vi "Create Ramp Buffer.vi"(8 "error in (no error)":errorcluster, 10 "initial value":u8, 11 "size":u64=1024) -> (0 "error out":errorcluster, 2 "buffer out":u8[](array[numeric]), 3 "pointer out":refnum<class "Memory.Pointer.Internal.lvclass">)   [LabVIEW 2016, in "Memory Manager Unit Tests.lvclass"]
uses:
  Memory Manager Unit Tests.lvclass
  Library/Classes/Pointer.Internal/Memory.Pointer.Internal.lvclass
  C:/Git/Personal/LabVIEW-Memory-Manager/Source/Library/Classes/Pointer/Memory.Pointer.lvclass
  Library/Classes/Pointer/Memory.Pointer.lvclass/Memory.Pointer.ctl
  Library/Classes/Pointer/Methods/Memory.Pointer.Write.Safe.1D.U8.vi
  Library/Classes/Pointer/Accessors/Set Address.vi
  Library/Classes/Pointer/Accessors/Set Size.vi
  Library/Classes/Pointer/Methods/Memory.Pointer.Write.Unsafe.1D.U8.vi
  Library/Classes/Pointer/Methods/Memory.Pointer.Parameter Check.Size.1D (Power of 2).vi
  Library/Classes/Pointer/Accessors/Get Address.vi
  Library/Classes/Pointer/Methods/Memory.Pointer.Errors.vi
  Library/Classes/Pointer/Methods/Memory.Pointer.Errors.Buffer Underflow.vi
  Library/Classes/Pointer/Methods/Memory.Pointer.Parameter Check.Size.0D.vi
  Library/Classes/Pointer/Methods/Memory.Pointer.Errors.Create Error.vi
  Submodules/Static Error Handling/Source/Library/VIs/Static Error Handling.Source Buffer.Write.String.vi
  Submodules/Static Error Handling/Source/Library/VIs/Static Error Handling.Source Buffer.Write.Numeric.Scalar.Base10.vi
  Submodules/Static Error Handling/Source/Library/VIs/Static Error Handling.Source Buffer.Write.Numeric.Scalar.Base10 (U64).vi
  Library/Classes/Pointer/Methods/Memory.Pointer.Errors.Out of Bounds.vi
  Library/Classes/Pointer/Accessors/Get Size.vi
  Submodules/Static Error Handling/Source/Library/VIs/Static Error Handling.Error Cluster Constant.vi
  Submodules/Static Error Handling/Source/Library/VIs/Static Error Handling.Error Cluster Constant (256B).vi
  Submodules/Static Error Handling/Source/Library/VIs/Static Error Handling.Parameters.Status.Set.vi
  Submodules/Static Error Handling/Source/Library/VIs/Static Error Handling.Parameters.Code.Set.vi
  Submodules/Static Error Handling/Source/Library/VIs/Static Error Handling.Parameters.VI Source.Set.vi
  Library/Constants/Memory.Constants.vi
  Library/Constants/Memory.Constants.Library Name.vi
  Library/Classes/Pointer/Methods/Memory.Pointer.Errors.Get Info.vi
  Library/Classes/Pointer/Methods/Memory.Pointer.Errors.Write Pointer Size.vi
  Library/Classes/Pointer/Memory.Pointer.lvclass
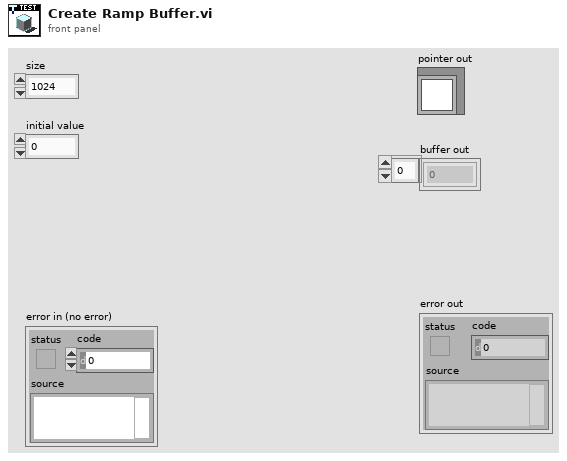
[diagram p1: front panel]
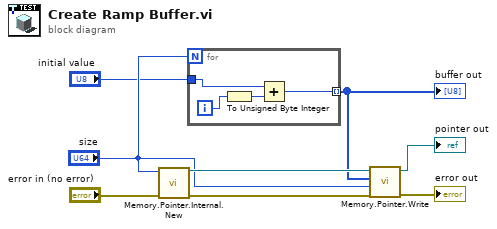
[diagram p0: block diagram]
diagram:
  n1 = call "Memory.Pointer.Internal.New.vi"("error in (no error)"="error in (no error)", "size"="size") -> ("error out"=w8:errorcluster, "pointer"=w7:refnum<class "Memory.Pointer.Internal.lvclass">)  [unwired: 8 in]
  n2 = for {
    N: "size" -> [_]
    tunnel: [w10] -> w5 mode=indexing
    tunnel: "initial value" -> [w9]
    i -> [w12]
    n3 = To Unsigned Byte Integer(number=w12) -> (unsigned 8bit integer=w11:u8)
    n4 = Add(x=w9, y=w11) -> (x+y=w10:u8)
  }
  "buffer out" <- w5
  n5 = call-poly "Memory.Pointer.Write.vi"("error in (no error)"=w8, "count"="size", "buffer in"=w5, "pointer in"=w7) -> ("error out"=→"error out":errorcluster, "pointer out"=→"pointer out":refnum<class "Memory.Pointer.Internal.lvclass">)  [unwired: 4 in, 2 out]
